vi "Unset Busy.vi"(8 "error in (no error)":errorcluster, 10 "VI reference (current VI)":refnum<vi>) -> (0 "error out":errorcluster)   [LabVIEW 2020]
doc: "Changes the appearance of the cursor on the front panel of a VI from a busy cursor to the default LabVIEW cursor and enables the mouse on the front panel."
uses:
  Set Cursor (Icon Pict).vi
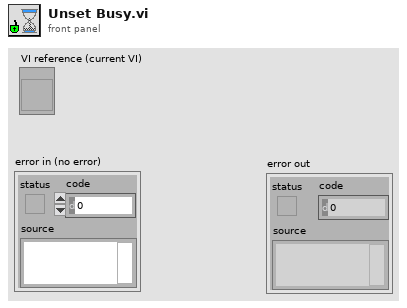
[diagram p1: front panel]
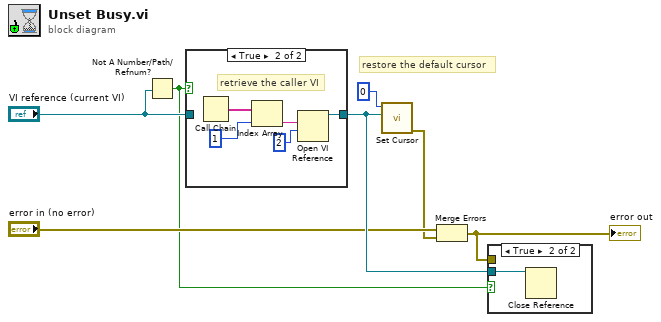
[diagram p0: block diagram]
diagram:
  # "restore the default cursor"
  n1 = Not A Number/Path/Refnum?(number/path/refnum="VI reference (current VI)") -> (NaN/Path/Refnum?=w1:bool)
  n2 = case shown="True" w1 {
    tunnel: [w8 w9] -> w6
    tunnel: "VI reference (current VI)" -> [w8 _]
    frame False {
    }
    frame True {
      # "retrieve the caller VI"
      n3 = Call Chain() -> (call chain=w12:string[])
      n4 = Index Array(array=w12, index=1) -> (element=w10:string)
      n5 = Open VI Reference(vi path=w10, options=2) -> (vi reference=w9:refnum<vi>)  [unwired: 4 in, 1 out]
    }
  }
  n6 = call-poly "Set Cursor.vi"("VI reference (current VI)"=w6, "icon"=u16 0 ("icons")) -> ("error out"=w3:errorcluster)  [unwired: 8 in, 1 out]
  n7 = Merge Errors("error in (no error)", w3) -> (w2:errorcluster)
  "error out" <- w2
  n8 = case shown="True" w1 {
    tunnel: w6 -> [_ w14]
    tunnel: w2 -> [_ _]
    frame False {
    }
    frame True {
      n9 = Close Reference(reference=w14) -> ()  [unwired: 1 in, 1 out]
    }
  }
